vi "gen_DAC_voltages.vi"(9 "counter cluster in":T2, 10 "scan specification":T3={"x amplitude"=0, "x resolution (pixels)"=0, "x offset fly-forward (iterations)"=0, "x offset fly-back (iterations)"=0, "y resolution (nr. of lines)"=0, "y step size"=0, "iterations per pixel"=0, "number of frames"=0, "y offset (pixels)"=0, "number of y-brake lines  (before y-fly-back)"=0, "number y-brake lines (after y-fly-back)"=0, "number of y-fly-back steps"=8, "lines per z step"=0, "number of z/intensity tuples"=0, "number of repetitions (volumes or planes)"=0}, 11 "resonant trigger":bool) -> (0 "galvo voltage in range?":bool, 1 "galvo moving forward?":bool, 2 "counter cluster out":T2, 3 "DAC voltages":T1 {"ch6" max=4095 step=1; "ch5" max=4095 step=1; "ch4" max=4095 step=1; "ch3" max=4095 step=1; "ch2" max=4095 step=1; "ch1" max=4095 step=1; "ch0" max=4095 step=1})   [LabVIEW 2010]
uses:
  counter_cluster.ctl
  scan_specification_cluster.ctl
  common_typedefs/DAC_voltage_cluster.ctl
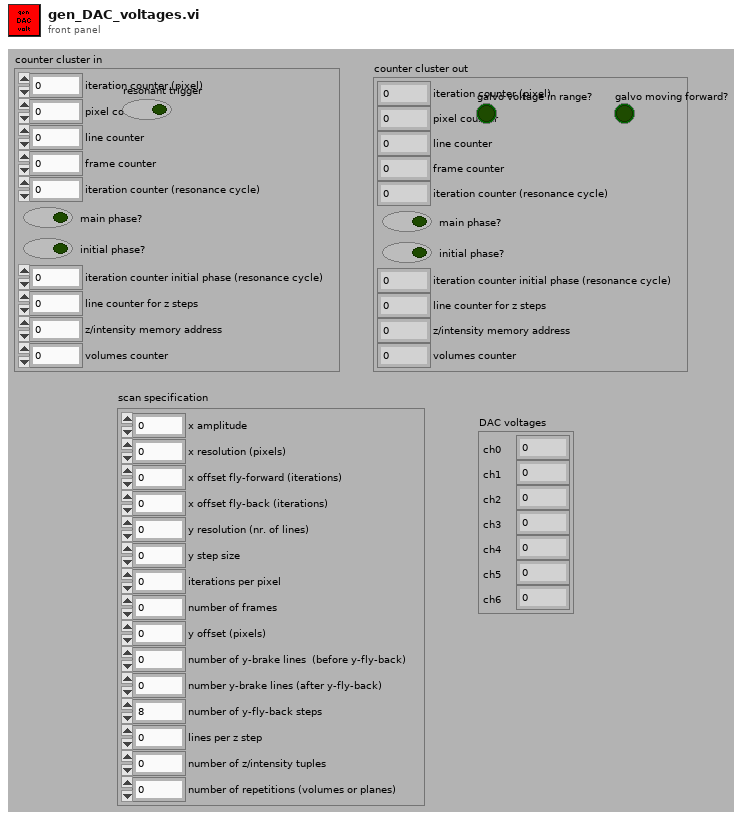
[diagram p1: front panel]
types:
  T1 = typedef "DAC_voltage_cluster.ctl" = cluster{"ch0":u16, "ch1":u16, "ch2":u16, "ch3":u16, "ch4":u16, "ch5":u16, "ch6":u16}
  T2 = typedef "counter_cluster.ctl" = cluster{"iteration counter (pixel)":u16, "pixel counter":u16, "line counter":u16, "frame counter":u16, "iteration counter (resonance cycle)":u16, "main phase?":bool, "initial phase?":bool, "iteration counter initial phase (resonance cycle)":u16, "line counter for z steps":u16, "z/intensity memory address":u32, "volumes counter":u16}
  T3 = typedef "scan_specification_cluster.ctl" = cluster{"x amplitude":u16, "x resolution (pixels)":u16, "x offset fly-forward (iterations)":u16, "x offset fly-back (iterations)":u16, "y resolution (nr. of lines)":u16, "y step size":u16, "iterations per pixel":u16, "number of frames":i32, "y offset (pixels)":u16, "number of y-brake lines  (before y-fly-back)":u16, "number y-brake lines (after y-fly-back)":u16, "number of y-fly-back steps":u16, "lines per z step":u16, "number of z/intensity tuples":u16, "number of repetitions (volumes or planes)":i32}
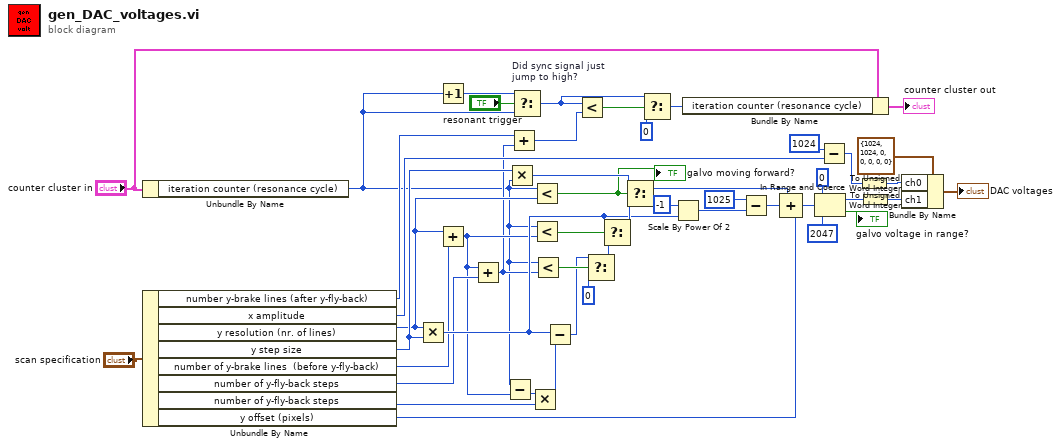
[diagram p0: block diagram]
diagram:
  n1 = Unbundle By Name("counter cluster in") -> ("iteration counter (resonance cycle)"=w6:u16)
  n2 = Unbundle By Name("scan specification") -> ("number y-brake lines (after y-fly-back)"=w12:u16, "x amplitude"=w14:u16, "y resolution (nr. of lines)"=w15:u16, "y step size"=w16:u16, "number of y-brake lines  (before y-fly-back)"=w22:u16, "number of y-fly-back steps"=w24:u16, "number of y-fly-back steps"=w23:u16, "y offset (pixels)"=w21:u16)
  n3 = Multiply(x=w15, y=w16) -> (x*y=w39:u16)
  n4 = Increment(x=w6) -> (x+1=w46:u16)
  n5 = Add(x=w15, y=w22) -> (x+y=w20:u16)
  n6 = Add(x=w20, y=w24) -> (x+y=w13:u16)
  n7 = Subtract(x=w6, y=w20) -> (x-y=w25:u16)
  n8 = Multiply(x=w16, y=w6) -> (x*y=w40:u16)
  n9 = Add(x=w12, y=w13) -> (x+y=w11:u16)
  n10 = Select "Did sync signal just\njump to high?"(t=w46, s="resonant trigger", f=w6) -> (s? t:f=w9:u16)
  n11 = Multiply(x=w25, y=w23) -> (x*y=w42:u16)
  n12 = Less?(x=w6, y=w15) -> (x < y?=w5:bool)
  "galvo moving forward?" <- w5
  n13 = Less?(x=w6, y=w20) -> (x < y?=w45:bool)
  n14 = Less?(x=w6, y=w13) -> (x < y?=w43:bool)
  n15 = Subtract(x=w39, y=w42) -> (x-y=w27:u16)
  n16 = Less?(x=w9, y=w11) -> (x < y?=w10:bool)
  n17 = Select(t=w27, s=w43, f=u16 0) -> (s? t:f=w41:u16)
  n18 = Select(t=w39, s=w45, f=w41) -> (s? t:f=w44:u16)
  n19 = Select(t=w40, s=w5, f=w44) -> (s? t:f=w18:u16)
  n20 = Select(t=w9, s=w10, f=u16 0) -> (s? t:f=w8:u16)
  n21 = Scale By Power Of 2(n=i16 -1, x=w39) -> (x*2^n=w38:u16)
  n22 = Bundle By Name(cluster="counter cluster in", "iteration counter (resonance cycle)"=w8) -> (→"counter cluster out":T2)
  n23 = Subtract(x=u16 1025, y=w38) -> (x-y=w17:u16)
  n24 = Compound Arithmetic op=ADD(w18, w17, w21) -> (w34:u16)
  n25 = In Range and Coerce(upper limit=u16 0, x=w34, lower limit=u16 2047) -> (coerced(x)=w1:u16, In Range?=→"galvo voltage in range?":bool)
  n26 = Subtract(x=u16 1024, y=w14) -> (x-y=w4:u16)
  n27 = To Unsigned Word Integer(number=w4) -> (unsigned 16bit integer=w3:u16)
  n28 = To Unsigned Word Integer(number=w1) -> (unsigned 16bit integer=w2:u16)
  n29 = Bundle By Name(cluster=T1 {"ch0"=1024, "ch1"=1024, "ch2"=0, "ch3"=0, "ch4"=0, "ch5"=0, "ch6"=0} ("DAC voltage"), "ch0"=w3, "ch1"=w2) -> (→"DAC voltages":T1)
